vi "TestCalibrationSetupEnd.vi"() -> ()   [LabVIEW 2019]
uses:
  enable_disable_enum_typedef.ctl
  MotorController.lvclass
panel:
  out "Error Out":errorcluster
  in  "Serial Port":refnum<visa-resource-name>
  in  "Error In":errorcluster
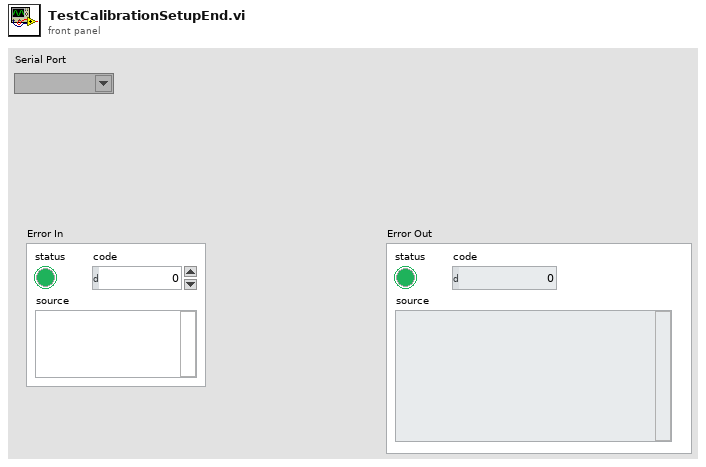
[diagram p1: front panel]
types:
  T1 = typedef "MotorController.lvclass/enable_disable_enum_typedef.ctl" = enum16{"Enable", "Disable"}
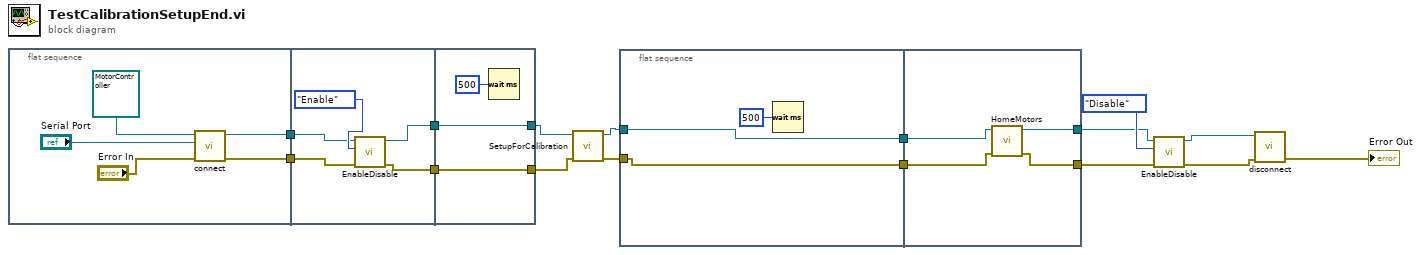
[diagram p0: block diagram]
diagram:
  n1 = flat-sequence {
    tunnel: [w19] -> w16
    tunnel: [w18] -> w15
    tunnel: w16 -> [w24]
    tunnel: w15 -> [w26]
    tunnel: [w23] -> w10
    tunnel: [w22] -> w9
    tunnel: [w28] -> w2
    tunnel: [w29] -> w1
    tunnel: w10 -> [w29]
    tunnel: w9 -> [w28]
    frame #0 {
      n2 = call "connect.vi"("error in (no error)"="Error In", "Serial Port"="Serial Port", "MotorController in"=refnum<class "MotorController.lvclass"> refnum ("MotorController.lvclass")) -> ("error out"=w18:errorcluster, "MotorController out"=w19:refnum<class "MotorController.lvclass">)  [unwired: 7 in]
    }
    frame #1 {
      n3 = call "EnableDisable.vi"("error in (no error)"=w26, "Action"=enable_disable_enum_typedef."Enable", "MotorController in"=w24) -> ("error out"=w23:errorcluster, "MotorController out"=w22:refnum<class "MotorController.lvclass">)  [unwired: 7 in]
    }
    frame #2 {
      n4 = Wait (ms)(milliseconds to wait=u32 500) -> ()  [unwired: 1 out]
    }
  }
  n5 = call "SetupForCalibration.vi"("Error In"=w1, "MotorController in"=w2) -> ("Error Out"=w3:errorcluster, "MotorController out"=w4:refnum<class "MotorController.lvclass">)  [unwired: 8 in]
  n6 = flat-sequence {
    tunnel: w4 -> [w31]
    tunnel: [w31] -> w8
    tunnel: [w30] -> w7
    tunnel: w3 -> [w30]
    tunnel: w8 -> [w36]
    tunnel: w7 -> [w35]
    tunnel: [w34] -> w6
    tunnel: [w33] -> w5
    frame #0 {
      n7 = Wait (ms)(milliseconds to wait=u32 500) -> ()  [unwired: 1 out]
    }
    frame #1 {
      n8 = call "HomeMotors.vi"("error in (no error)"=w35, "MotorController in"=w36) -> ("error out"=w34:errorcluster, "MotorController out"=w33:refnum<class "MotorController.lvclass">)  [unwired: 8 in]
    }
  }
  n9 = call "EnableDisable.vi"("error in (no error)"=w6, "Action"=enable_disable_enum_typedef."Disable", "MotorController in"=w5) -> ("error out"=w11:errorcluster, "MotorController out"=w12:refnum<class "MotorController.lvclass">)  [unwired: 7 in]
  n10 = call "disconnect.vi"("error in (no error)"=w11, "MotorController in"=w12) -> ("error out"=→"Error Out":errorcluster)  [unwired: 8 in, 1 out]
